vi "Find Value.vi"(7 "Type":refnum<class>, 8 "error in (no error)":errorcluster, 10 "Path":string, 11 "PathTree in":refnum<class "PathTree.lvclass">) -> (0 "error out":errorcluster, 2 "Value":refnum<class>, 3 "PathTree out":refnum<class "PathTree.lvclass">)   [LabVIEW 2020, in "Advanced Structures.lvlib" / "PathTree.lvclass"]
uses:
  PathTree.lvclass
  PathTreeNode/PathTreeNode.lvclass
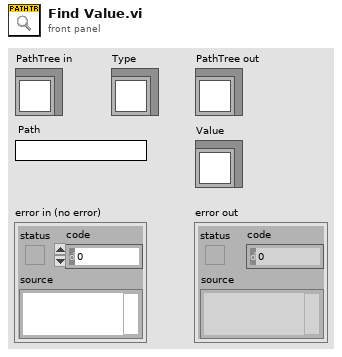
[diagram p1: front panel]
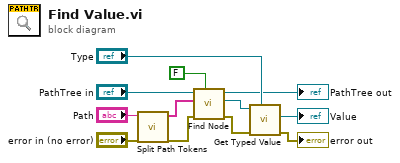
[diagram p0: block diagram]
diagram:
  n1 = call "Split Path Tokens.vi"("Path"="Path") -> ("Tokens"=w9:string[])  [unwired: 10 in]
  n2 = call "Find Node.vi"("Create?"=FALSE, "error in (no error)"="error in (no error)", "Tokens"=w9, "PathTree in"="PathTree in") -> ("error out"=w3:errorcluster, "Node"=w8:refnum<class "PathTreeNode.lvclass">, "PathTree out"=→"PathTree out":refnum<class "PathTree.lvclass">)  [unwired: 5 in]
  n3 = call "Get Typed Value.vi"("Type"="Type", "error in (no error)"=w3, "PathTreeNode in"=w8) -> ("error out"=→"error out":errorcluster, "Typed Value"=→"Value":refnum<class>)  [unwired: 6 in, 1 out]
